vi "SMS Image Preview.vi"(7 "Calling VI Ref":refnum<vi>) -> ()   [LabVIEW 2020]
uses:
  <vilib>/Utility/miscctls.llb/LVPointTypeDef.ctl
  Hardware Configuration/Hardware Configuration Controls/Device Function.ctl
  SMS Image Preview Type Defs/SMS Image Preview Notifier Type.ctl
  SMS Image Preview Type Defs/SMS Image Preview Actions.ctl
  <vilib>/vision/Image Controls.llb/IMAQ Image.ctl
  Device Library/Cameras/Hamamatsu/Orca Flash/Orca Flash Controls/Orca Flash Actions.ctl
  Hardware Configuration/Hardware Configuration Controls/Device Type.ctl
  Device Library/Cameras/Camera Controls/Camera IMAQ Key Info.ctl
  <vilib>/vision/NI_Vision_Development_Module.lvlib
panel:
  in  "Reset Plot":bool
  out "Blink No. vs. Time":cluster{dbl[], u16[]}(graph)
  in  "Accumulate":bool
  in  "Blink Sensitivity":sgl=1.3
  in  "Image Display":bool
  in  "SMS Preview":bool
  in  "Camera ROI":bool
  in  "Camera":i32(ring) items=["Hamamatsu-Camera-Primary-0"]
  in  "Quit":bool
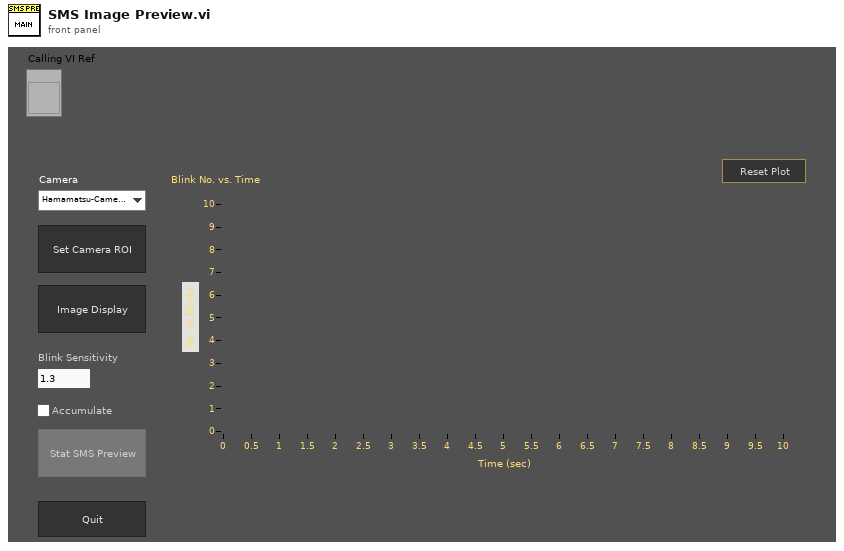
[diagram p1: front panel]
types:
  T1 = typedef "Orca Flash Actions.ctl" = enum16{"Idle", "Preview", "Record", "Record Settings", "Set Param", "Get Param", "Set ROI", "Get ROI", "Trigger Source", "Trigger Type", "Progessive Mode", "Area Mode", "Status", "Quit"}
  T2 = enum8{"Enabled", "Disabled", "Disabled and Grayed Out"}
  T3 = typedef "SMS Image Preview Actions.ctl" = enum16{"Idle", "Start SMS Preview", "Get Image", "Convolve and Threshold", "Subtract > Dilate", "And Image", "Update Plot", "Abort", "Exit Loop", "Quit"}
  T4 = typedef "SMS Image Preview Notifier Type.ctl" = cluster{"Action":T3, "Camera Notifier Name":string, "Camera Image (U16)":T5, "Camera ROI":cluster{"Global Rectangle":i32[], "Contours":cluster{"Contour Type":u32, "ROI Type":u32, "Points":i32[]}[]}, "SMS Preview (U16)":T5, "Camera ROI (U16)":T5, "Threshold (U16)":T5, "Subtracted > Dilated (U16)":T5, "And Image (U16)":T5, "Camera ROI (SGL)":T5, "Conv 5 x 5 (SGL)":T5, "Conv 11 x 11 (SGL)":T5, "Subtracted (SGL)":T5, "Dilated (SGL)":T5, "Subtracted > Dilated (SGL)":T5, "Ones 5 x 5":sgl[][], "Ones 11 x 11":sgl[][], "Ones 7 x 7":i32[][]}
  T5 = typedef "IMAQ Image.ctl" = refnum<image>
  T6 = typedef "Device Function.ctl" = enum16{"Primary", "Secondary", "Overview", "Wide Field Drift Correction", "642 nm Excitation", "560 nm Excitation", "940 nm Excitation", "546 nm Excitation", "488 nm Excitation", "405 nm Excitation", "Objective Drift Correction", "4Pi Objective Lock", "Objective XY", "Objective Z", "Sample XY", "Sample Coarse Z", "Sample Z", "4Pi Lower", "4Pi Upper", "Mojo", "Adj Cavity", "Line Scanning", "Alert"}
  T7 = enum16{"Always On", "Always Off", "Off While Running"}
  T8 = typedef "LVPointTypeDef.ctl" = cluster{"Horizontal":i16, "Vertical":i16}
  T9 = typedef "Image Type" = u32
  T10 = typedef "Device Type.ctl" = enum16{"AOTF", "Camera", "Deformable Mirror", "Laser", "Microscope Base", "Shutter", "Stage", "Waveform", "FPGA", "Email", "Filter Wheel", "Spinning Disk"}
  T11 = typedef "Camera IMAQ Key Info.ctl" = cluster{"Frame":u32, "Sensor Height":i32, "Sensor Width":i32, "ROI Height":i32, "ROI Width":i32, "ROI Enable?":bool, "Bit per Pixel":u8}
  T12 = enum32{"Average", "Min", "Max", "Clear  if < ", "Clear  if < or =", "Clear  if =", "Clear  if > or =", "Clear  if >"}
  T13 = enum32{"AutoM", "Close", "Dilate", "Erode", "Gradient", "Gradient in", "Gradient out", "HitMiss", "Open", "PClose", "POpen", "Thick", "Thin"}
  T14 = enum32{"Invalid", "Standard", "Closed", "Hidden", "Minimized", "Maximized"}
  T15 = cluster{"Global Rectangle":i32[], "Contours":cluster{"Contour Type":u32, "ROI Type":u32, "Points":i32[]}[]}
  T16 = cluster{"histogram":u32[], "Minimal Value":sgl, "Maximal Value":sgl, "Starting Value":sgl, "Interval Width":sgl, "Mean Value":sgl, "Standard  Variation":sgl, "Area (pixels)":i32}
  T17 = typedef "LVRectTypeDef.ctl" = cluster{"Left":i16, "Top":i16, "Right":i16, "Bottom":i16}
  T18 = typedef "LVBoundsTypeDef.ctl" = cluster{"Width":u32, "Height":u32}
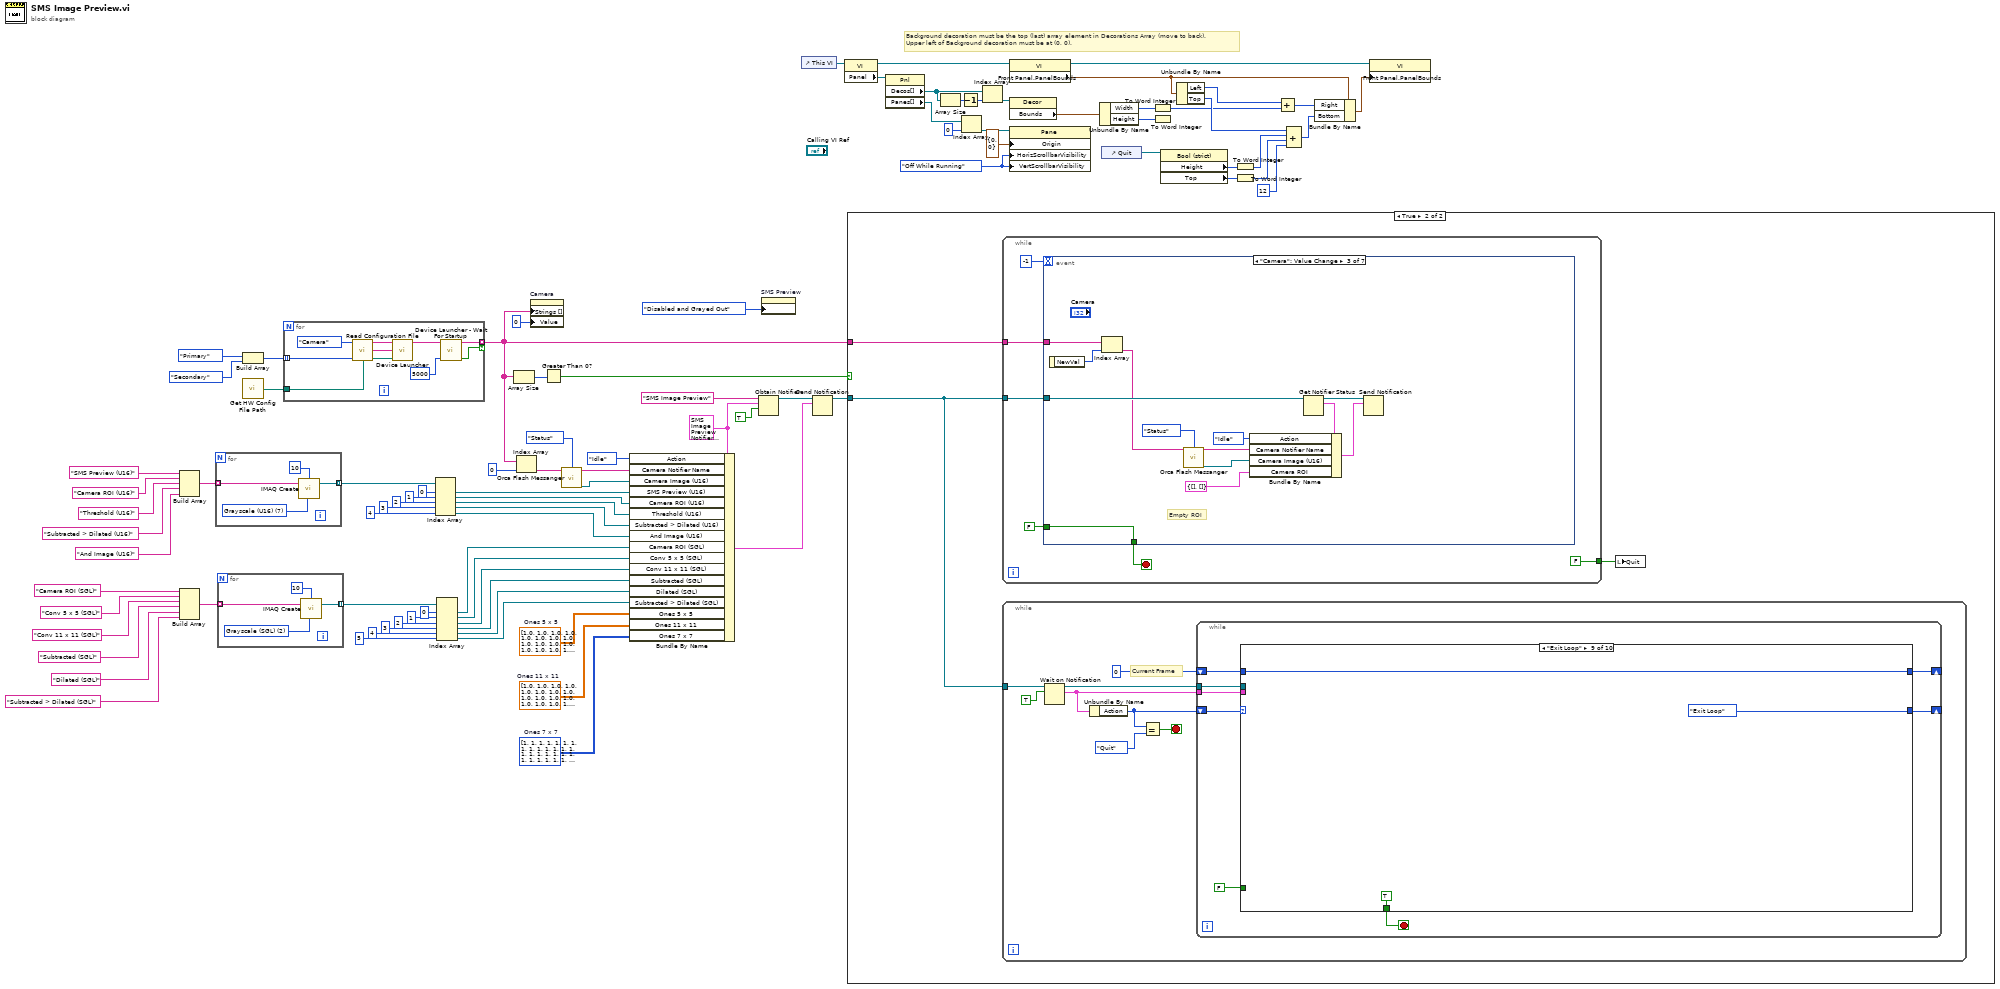
[diagram p0: block diagram]
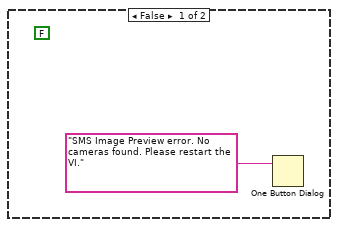
[diagram p2: hidden frame]
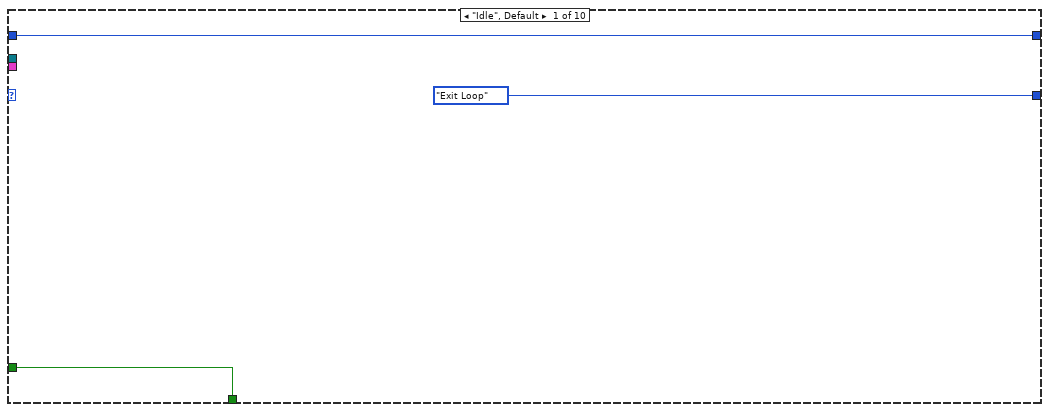
[diagram p3: hidden frame]
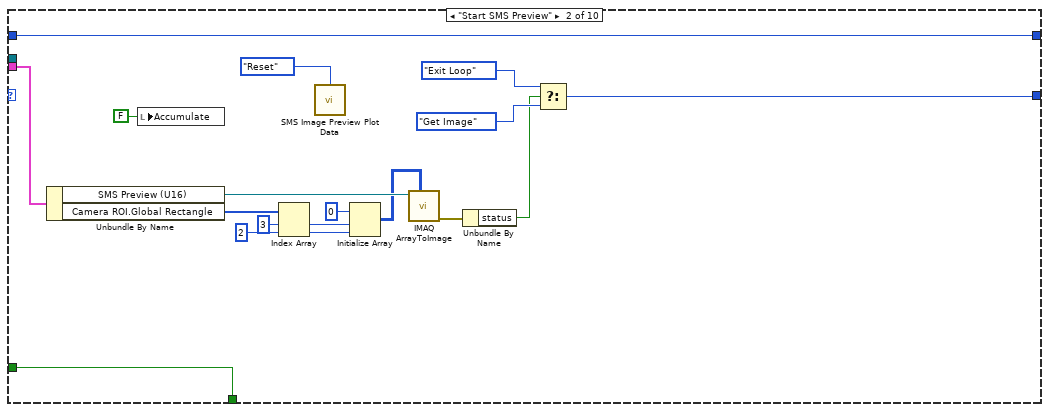
[diagram p4: hidden frame]
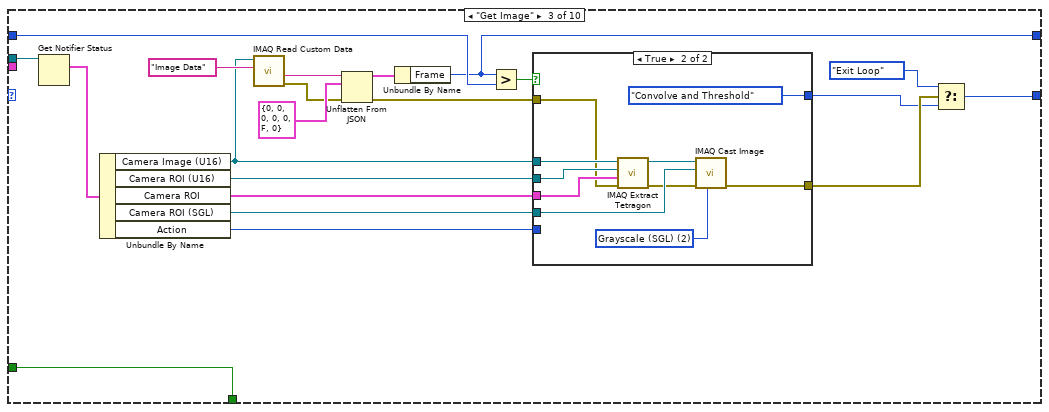
[diagram p5: hidden frame]
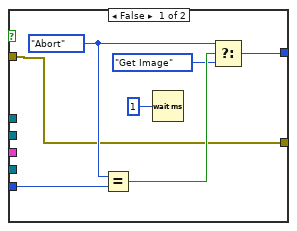
[diagram p6: hidden frame]
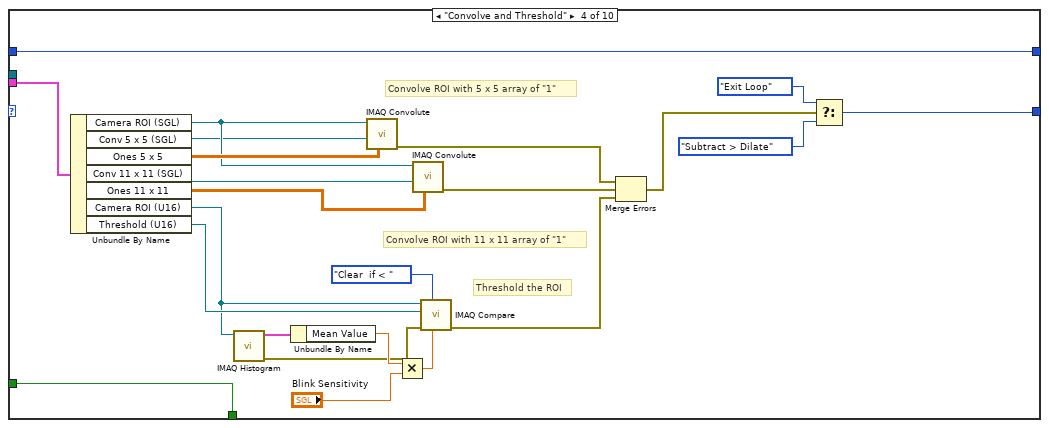
[diagram p7: hidden frame]
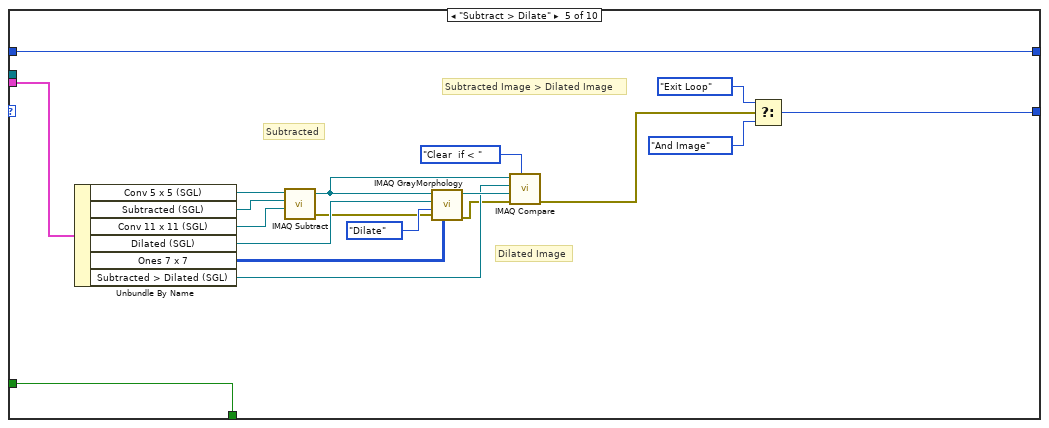
[diagram p8: hidden frame]
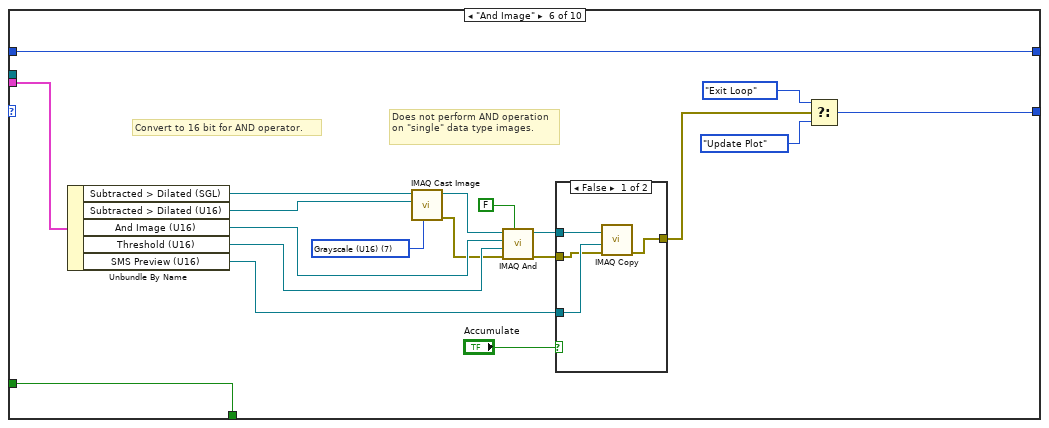
[diagram p9: hidden frame]
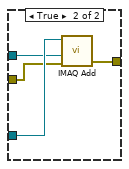
[diagram p10: hidden frame]
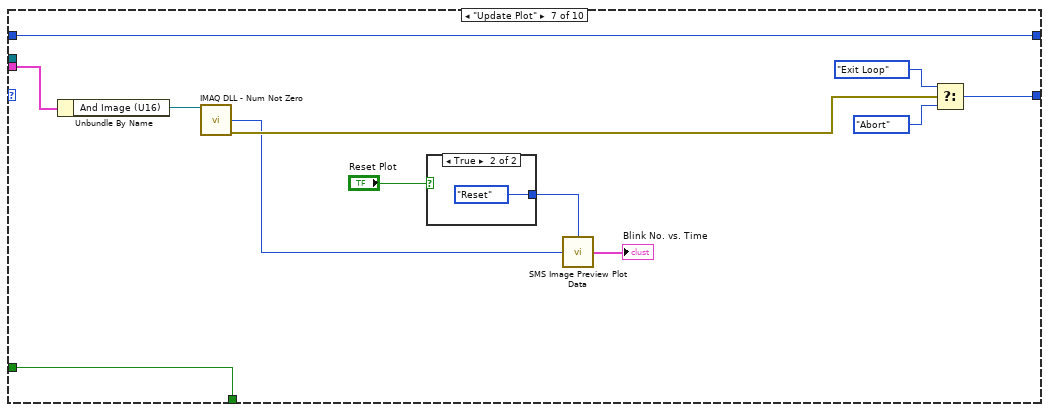
[diagram p11: hidden frame]
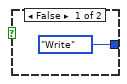
[diagram p12: hidden frame]
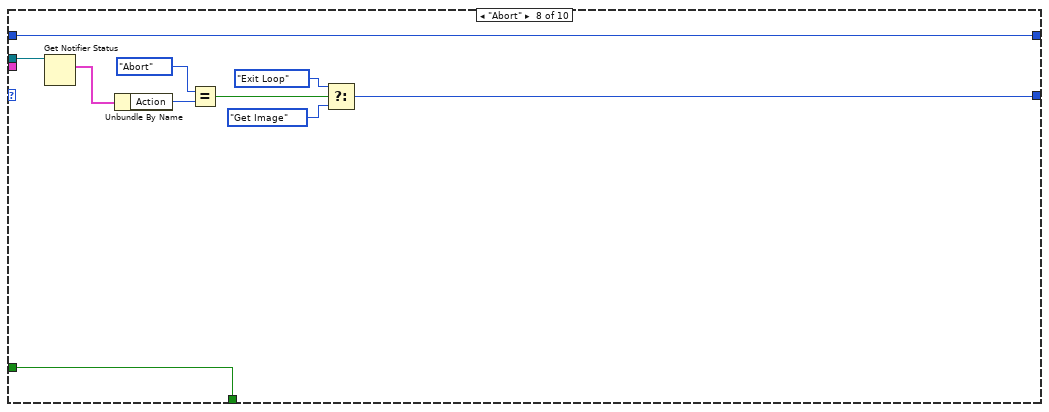
[diagram p13: hidden frame]
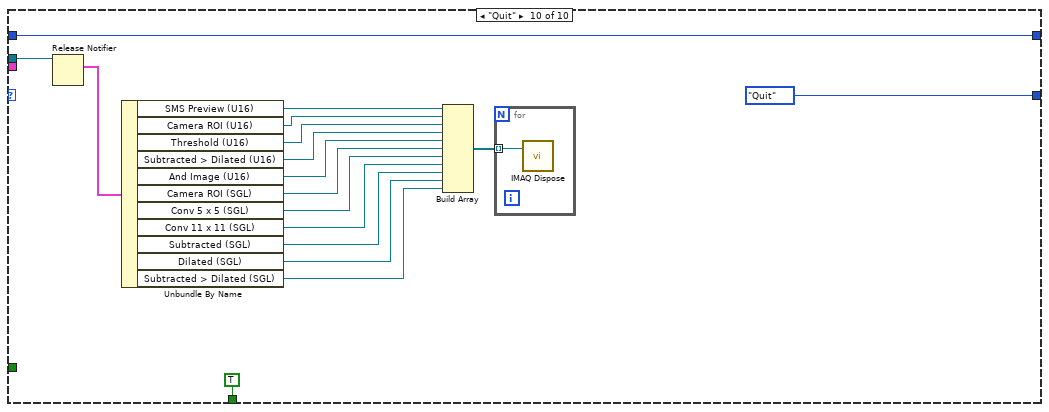
[diagram p14: hidden frame]
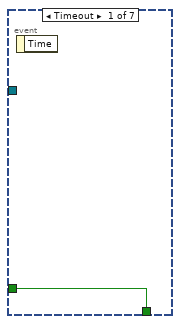
[diagram p15: hidden frame]
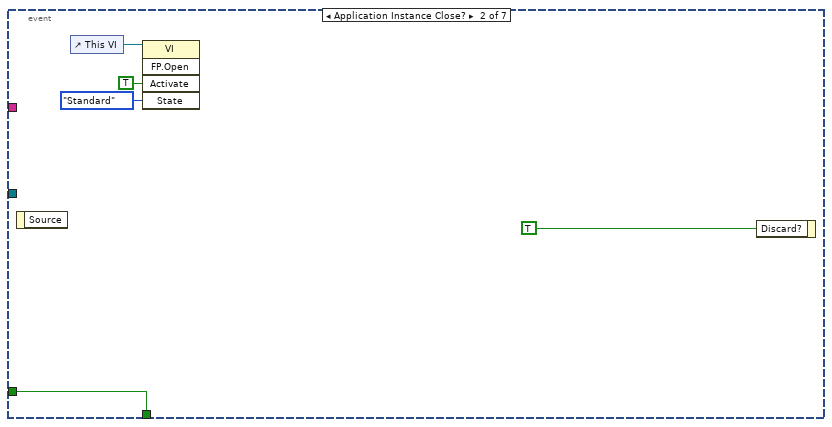
[diagram p16: hidden frame]
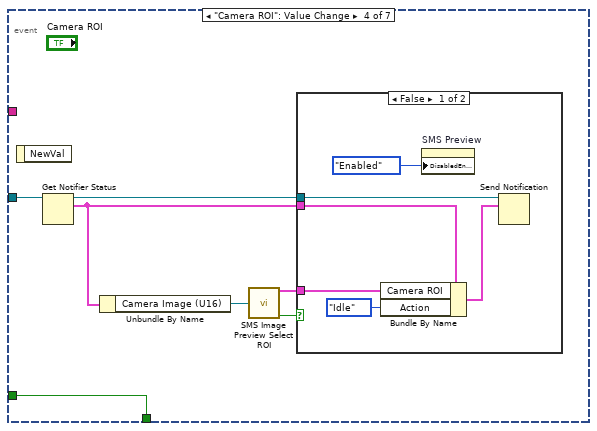
[diagram p17: hidden frame]
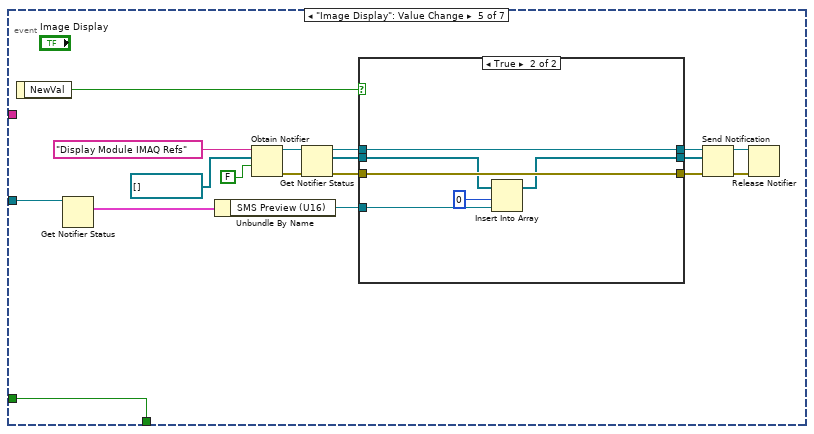
[diagram p19: hidden frame]
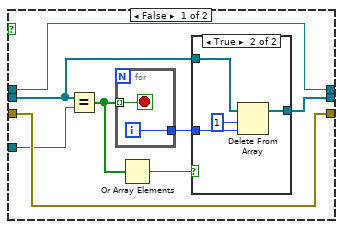
[diagram p20: hidden frame]
diagram:
  w3 = i32[][] [[1, 1, 1, 1, 1, 1, 1], [1, 1, 1, 1, 1, 1, 1], [1, 1, 1, 1, 1, 1, 1], [1, 1, 1, 1, 1, 1, 1], [1, 1, 1, 1, 1, 1, 1], [1, 1, 1, 1, 1, 1, 1], [1, 1, 1, 1, 1, 1, 1]]  # Ones 7 x 7
  w4 = sgl[][] [[1.0, 1.0, 1.0, 1.0, 1.0, 1.0, 1.0, 1.0, 1.0, 1.0, 1.0], [1.0, 1.0, 1.0, 1.0, 1.0, 1.0, 1.0, 1.0, 1.0, 1.0, 1.0], [1.0, 1.0, 1.0, 1.0, 1.0, 1.0, 1.0, 1.0, 1.0, 1.0, 1.0], [1.0, 1.0, 1.0, 1.0, 1.0, 1.0, 1.0, 1.0, 1.0, 1.0, 1.0], [1.0, 1.0, 1.0, 1.0, 1.0, 1.0, 1.0, 1.0, 1.0, 1.0, 1.0], [1.0, 1.0, 1.0, 1.0, 1.0, 1.0, 1.0, 1.0, 1.0, 1.0, 1.0], [1.0, 1.0, 1.0, 1.0, 1.0, 1.0, 1.0, 1.0, 1.0, 1.0, 1.0], [1.0, 1.0, 1.0, 1.0, 1.0, 1.0, 1.0, 1.0, 1.0, 1.0, 1.0], [1.0, 1.0, 1.0, 1.0, 1.0, 1.0, 1.0, 1.0, 1.0, 1.0, 1.0], [1.0, 1.0, 1.0, 1.0, 1.0, 1.0, 1.0, 1.0, 1.0, 1.0, 1.0], [1.0, 1.0, 1.0, 1.0, 1.0, 1.0, 1.0, 1.0, 1.0, 1.0, 1.0]]  # Ones 11 x 11
  w5 = sgl[][] [[1.0, 1.0, 1.0, 1.0, 1.0], [1.0, 1.0, 1.0, 1.0, 1.0], [1.0, 1.0, 1.0, 1.0, 1.0], [1.0, 1.0, 1.0, 1.0, 1.0], [1.0, 1.0, 1.0, 1.0, 1.0]]  # Ones 5 x 5
  w51 = T4 {"Action"=enum."Idle", "Camera Notifier Name"="", "Camera Image (U16)"=refnum, "Camera ROI"={"Global Rectangle"=[], "Contours"=[]}, "SMS Preview (U16)"=refnum, "Camera ROI (U16)"=refnum, "Threshold (U16)"=refnum, "Subtracted > Dilated (U16)"=refnum, "And Image (U16)"=refnum, "Camera ROI (SGL)"=refnum, "Conv 5 x 5 (SGL)"=refnum, "Conv 11 x 11 (SGL)"=refnum, "Subtracted (SGL)"=refnum, "Dilated (SGL)"=refnum, "Subtracted > Dilated (SGL)"=refnum, "Ones 5 x 5"=[], "Ones 11 x 11"=[], "Ones 7 x 7"=[]} ("SMS Image Preview Notifier Type")
  w73 = T7."Off While Running" ("Vertical Scrollbar Visibility")
  # "Background decoration must be the top (last) array element in Decorations Array (move to back).\nUpper left of Background decoration must be at (0, 0)."
  n1 = Build Array("Camera ROI (SGL)" ("Image Name"), "Conv 5 x 5 (SGL)" ("Image Name"), "Conv 11 x 11 (SGL)" ("Image Name"), "Subtracted (SGL)" ("Image Name"), "Dilated (SGL)" ("Image Name"), "Subtracted > Dilated (SGL)" ("Image Name")) -> (w37:string[])
  n2 = Build Array("SMS Preview (U16)" ("Image Name"), "Camera ROI (U16)" ("Image Name"), "Threshold (U16)" ("Image Name"), "Subtracted > Dilated (U16)" ("Image Name"), "And Image (U16)" ("Image Name")) -> (w17:string[])
  n3 = for {
    tunnel: w17 -> [w92] mode=indexing
    tunnel: [w91] -> w18 mode=indexing
    w93 = T9 7 items=["Grayscale (U8)", "Grayscale (I16)", "Grayscale (SGL)", "Complex (CSG)", "RGB (U32)", "HSL (U32)", "RGB (U64)", "Grayscale (U16)"] ("Image Type")
    n4 = call "IMAQ Create"("Border Size"=10, "Image Name"=w92, "Image Type"=w93) -> ("New Image"=w91:T5)  [unwired: 2 in, 1 out]
  }
  n5 = for {
    tunnel: w37 -> [w96] mode=indexing
    tunnel: [w95] -> w36 mode=indexing
    w97 = T9 2 items=["Grayscale (U8)", "Grayscale (I16)", "Grayscale (SGL)", "Complex (CSG)", "RGB (U32)", "HSL (U32)", "RGB (U64)", "Grayscale (U16)"] ("Image Type")
    n6 = call "IMAQ Create"("Border Size"=10, "Image Name"=w96, "Image Type"=w97) -> ("New Image"=w95:T5)  [unwired: 2 in, 1 out]
  }
  n7 = Build Array(Device_Function."Primary" ("Device Function"), Device_Function."Secondary" ("Device Function")) -> (w59:T6[])
  n8 = call "Get HW Config File Path.vi"() -> ("File Path"=w58:path)  [unwired: 14 in, 1 out]
  n9 = for {
    tunnel: w59 -> [w104] mode=indexing
    tunnel: w58 -> [w103]
    tunnel: [w101] -> w47 mode=indexing if=w100
    n10 = call "Read Configuration File.vi"("Device Type"=Device_Type."Camera", "Device Function"=w104, "Config File Path"=w103) -> ("Unique Notifier Name"=w106:string, "Device Ports/IDs/Channels"=w108:string[], "Device Engine Path"=w107:path)  [unwired: 9 in, 1 out]
    n11 = call "Device Launcher.vi"("Notifier Name"=w106, "Device Ports/IDs/Channels"=w108, "Device Engine Path"=w107) -> ("Notifier Name"=w102:string)  [unwired: 11 in, 1 out]
    n12 = call "Device Launcher - Wait For Startup.vi"("Notifier Name"=w102, "Wait Time (ms)"=5000) -> ("Notifier Name (Dup)"=w101:string, "Running?"=w100:bool)  [unwired: 12 in]
  }
  n13 = Index Array(array=w18, index #1=0 ("index"), index #2=1 ("index"), index #3=2 ("index"), index #4=3 ("index"), index #5=4 ("index")) -> (element #1=w16:T5, element #2=w15:T5, element #3=w14:T5, element #4=w13:T5, element #5=w12:T5)
  n14 = Index Array(array=w36, index #1=0 ("index"), index #2=1 ("index"), index #3=2 ("index"), index #4=3 ("index"), index #5=4 ("index"), index #6=5 ("index")) -> (element #1=w11:T5, element #2=w10:T5, element #3=w9:T5, element #4=w8:T5, element #5=w7:T5, element #6=w6:T5)
  n15 = Array Size(array=w47) -> (size(s)=w57:i32)
  n16 = Index Array(array=w47, index=0) -> (element=w45:string)
  n17 = property on="Camera" class="Ring (strict)"("Strings []"=w47, "Value"=0) -> ()  [unwired: 2 in, 2 out]
  n18 = Greater Than 0?(x=w57) -> (x > 0?=w56:bool)
  n19 = call "Orca Flash Messanger.vi"("Notifier Name"=w45, "Camera Actions"=Orca_Flash_Actions."Status") -> ("Notifier Name Dup"=w44:string, "Image Ref"=w43:T5)  [unwired: 9 in, 3 out]
  n20 = Bundle By Name(cluster=w51, "Action"=SMS_Image_Preview_Actions."Idle", "Camera Notifier Name"=w44, "Camera Image (U16)"=w43, "SMS Preview (U16)"=w16, "Camera ROI (U16)"=w15, "Threshold (U16)"=w14, "Subtracted > Dilated (U16)"=w13, "And Image (U16)"=w12, "Camera ROI (SGL)"=w11, "Conv 5 x 5 (SGL)"=w10, "Conv 11 x 11 (SGL)"=w9, "Subtracted (SGL)"=w8, "Dilated (SGL)"=w7, "Subtracted > Dilated (SGL)"=w6, "Ones 5 x 5"=w5, "Ones 11 x 11"=w4, "Ones 7 x 7"=w3) -> (w48:T4)
  n21 = Obtain Notifier(name (unnamed)="SMS Image Preview", notification data type=w51, create if not found? (T)=TRUE) -> (notifier out=w52:refnum<notifier>)  [unwired: 1 in, 2 out]
  n22 = property on="SMS Preview" class="Bool (strict)"("DisabledEnum"=T2."Disabled and Grayed Out" ("Disabled")) -> ()  [unwired: 2 in, 2 out]
  n23 = control-ref of="This VI"() -> (w65:refnum<vi>)
  n24 = Send Notification(notification=w48, notifier=w52) -> (notifier out=w49:refnum<notifier>)  [unwired: 1 in, 1 out]
  n25 = property class="VI"(reference=w65) -> (reference out=w74:refnum<vi>, "Panel"=w66:refnum<vi>)  [unwired: 1 in, 1 out]
  n26 = case shown="True" w56 {
    tunnel: w47 -> [_ w112]
    tunnel: w49 -> [_ w110]
    frame False {
      (unwired) FALSE
      n27 = One Button Dialog(message="SMS Image Preview error. No cameras found. Please restart the VI.") -> ()  [unwired: 1 in, 1 out]
    }
    frame True {
      n28 = while {
        tunnel: w112 -> [w304]
        tunnel: w110 -> [w303]
        tunnel: [FALSE] -> w111
        stop <- w305 stop-if-true
        n29 = event shown="[2] \"Camera\": Value Change" {
          selector: _ -> [_ _ _ _ _ _ _]
          dyn-events: _ -> [_ _ _ _ _ _ _]
          timeout: -1 -> [_ _ _ _ _ _ _]
          tunnel: FALSE -> [w308 w312 w326 w333 w357 w387 _]
          tunnel: [w308 w312 w326 w333 w357 w387 w393] -> w305
          tunnel: w304 -> [_ _ w325 _ _ _ _]
          tunnel: w303 -> [_ _ w323 w332 w341 w386 w392]
          event Timeout {
            n30 = event-data() -> ()  [unwired: 1 in, 1 out]
          }
          event Application Instance Close? {
            n31 = event-data() -> ()  [unwired: 1 in, 1 out]
            n32 = control-ref of="This VI"() -> (w309:refnum<vi>)
            n33 = invoke class="VI" method="FP.Open"(reference=w309, "Activate"=TRUE ("Activate?"), "State"=T14."Standard") -> ()  [unwired: 2 in, 5 out]
            n34 = event-data("Discard?"=TRUE) -> ()  [unwired: 1 in, 1 out]
          }
          event "Camera": Value Change {
            # "Empty ROI"
            n35 = event-data() -> ("NewVal"=w324:i32)  [unwired: 1 in]
            n36 = Index Array(array=w325, index=w324) -> (element=w317:string)
            n37 = call "Orca Flash Messanger.vi"("Notifier Name"=w317, "Camera Actions"=Orca_Flash_Actions."Status") -> ("Notifier Name Dup"=w319:string, "Image Ref"=w318:T5)  [unwired: 9 in, 3 out]
            n38 = Get Notifier Status(notifier=w323) -> (notifier out=w322:refnum<notifier>, current notification=w321:T4)  [unwired: 1 in, 3 out]
            n39 = Bundle By Name(cluster=w321, "Action"=SMS_Image_Preview_Actions."Idle", "Camera Notifier Name"=w319, "Camera Image (U16)"=w318, "Camera ROI"=T15 {"Global Rectangle"=[], "Contours"=[]}) -> (w320:T4)
            n40 = Send Notification(notification=w320, notifier=w322) -> ()  [unwired: 1 in, 2 out]
          }
          event "Camera ROI": Value Change {
            n41 = event-data() -> ()  [unwired: 1 in, 1 out]
            n42 = Get Notifier Status(notifier=w332) -> (notifier out=w331:refnum<notifier>, current notification=w327:T4)  [unwired: 1 in, 3 out]
            n43 = Unbundle By Name(w327) -> ("Camera Image (U16)"=w330:T5)
            n44 = call "SMS Image Preview Select ROI.vi"("Camera Image Ref"=w330) -> ("Camera ROI"=w328:T15, "Canceled?"=w329:bool)  [unwired: 13 in]
            n45 = case shown="False" w329 {
              tunnel: w331 -> [w339 _]
              tunnel: w328 -> [w337 _]
              tunnel: w327 -> [w338 _]
              frame False {
                n46 = Bundle By Name(cluster=w338, "Camera ROI"=w337, "Action"=SMS_Image_Preview_Actions."Idle") -> (w336:T4)
                n47 = property on="SMS Preview" class="Bool (strict)"("DisabledEnum"=T2."Enabled" ("Disabled")) -> ()  [unwired: 2 in, 2 out]
                n48 = Send Notification(notification=w336, notifier=w339) -> ()  [unwired: 1 in, 2 out]
              }
              frame True {
              }
            }
          }
          event "Image Display": Value Change {
            n49 = event-data() -> ("NewVal"=w340:bool)  [unwired: 1 in]
            n50 = Get Notifier Status(notifier=w341) -> (current notification=w342:T4)  [unwired: 1 in, 4 out]
            n51 = Unbundle By Name(w342) -> ("SMS Preview (U16)"=w356:T5)
            n52 = Obtain Notifier(name (unnamed)="Display Module IMAQ Refs", notification data type=T5[] [], create if not found? (T)=FALSE) -> (notifier out=w349:refnum<notifier>, error out=w350:errorcluster)  [unwired: 1 in, 1 out]
            n53 = Get Notifier Status(notifier=w349, error in (no error)=w350) -> (notifier out=w348:refnum<notifier>, current notification=w346:T5[], error out=w347:errorcluster)  [unwired: 2 out]
            n54 = case shown="True" w340 {
              tunnel: w348 -> [w365 w378]
              tunnel: w347 -> [w359 w377]
              tunnel: w346 -> [w361 w376]
              tunnel: [w360 w373] -> w343
              tunnel: [w365 w378] -> w345
              tunnel: [w359 w377] -> w344
              tunnel: w356 -> [w358 w375]
              frame False {
                n55 = Equal?(x=w361, y=w358) -> (x = y?=w364:bool[])
                n56 = for {
                  tunnel: w364 -> [w372] mode=indexing
                  tunnel: [w371] -> w362
                  i -> [w371]
                  stop <- w372 stop-if-true
                }
                n57 = Or Array Elements(Boolean array=w364) -> (logical OR=w363:bool)
                n58 = case shown="True" w363 {
                  tunnel: w362 -> [_ w369]
                  tunnel: w361 -> [w366 w368]
                  tunnel: [w366 w367] -> w360
                  frame False {
                  }
                  frame True {
                    n59 = Delete From Array(array=w368, length=1, index=w369) -> (array with subset deleted=w367:T5[])  [unwired: 1 out]
                  }
                }
              }
              frame True {
                n60 = Insert Into Array(array=w376, index=0, new element=w375) -> (w373:T5[])
              }
            }
            n61 = Send Notification(notification=w343, notifier=w345, error in (no error)=w344) -> (notifier out=w351:refnum<notifier>, error out=w352:errorcluster)
            n62 = Release Notifier(notifier=w351, error in (no error)=w352) -> ()  [unwired: 1 in, 3 out]
          }
          event "SMS Preview": Value Change {
            n63 = event-data() -> ("NewVal"=w382:bool)  [unwired: 1 in]
            n64 = Get Notifier Status(notifier=w386) -> (notifier out=w385:refnum<notifier>, current notification=w384:T4)  [unwired: 1 in, 3 out]
            n65 = Select(t=SMS_Image_Preview_Actions."Start SMS Preview" ("Action"), s=w382, f=SMS_Image_Preview_Actions."Abort") -> (s? t:f=w379:T3)
            n66 = Bundle By Name(cluster=w384, "Action"=w379) -> (w383:T4)
            n67 = Send Notification(notification=w383, notifier=w385) -> ()  [unwired: 1 in, 2 out]
          }
          event "Quit": Value Change {
            n68 = event-data() -> ("NewVal"=w393:bool)  [unwired: 1 in]
            n69 = Get Notifier Status(notifier=w392) -> (notifier out=w390:refnum<notifier>, current notification=w389:T4)  [unwired: 1 in, 3 out]
            n70 = Bundle By Name(cluster=w389, "Action"=SMS_Image_Preview_Actions."Quit") -> (w391:T4)
            n71 = Send Notification(notification=w391, notifier=w390) -> ()  [unwired: 1 in, 2 out]
          }
        }
      }
      n72 = while {
        tunnel: w110 -> [w120]
        stop <- w117 stop-if-true
        # "Current Frame"
        n73 = Wait on Notification(notifier=w120, ignore previous (F)=TRUE) -> (notifier out=w113:refnum<notifier>, notification=w115:T4)  [unwired: 2 in, 2 out]
        n74 = Unbundle By Name(w115) -> ("Action"=w116:T3)
        n75 = Equal?(x=w116, y=SMS_Image_Preview_Actions."Quit") -> (x = y?=w117:bool)
        n76 = while {
          shift-right: [w126] -> _
          shift-left: w116 -> [w128]
          tunnel: w115 -> [w127]
          shift-right: [w124] -> _
          shift-left: u32 0 -> [w125]
          tunnel: w113 -> [w123]
          stop <- w121 stop-if-true
          n77 = case shown="\"Exit Loop\"" w128 {
            tunnel: w127 -> [_ w147 _ w209 w228 w247 w263 _ _ _]
            tunnel: [SMS_Image_Preview_Actions."Exit Loop" ("y") w136 w151 w190 w211 w230 w266 w274 SMS_Image_Preview_Actions."Exit Loop" ("f") SMS_Image_Preview_Actions."Quit" ("f")] -> w126
            tunnel: w125 -> [w130 w149 w166 w210 w229 w248 w267 w280 w283 w300]
            tunnel: [w130 w149 w165 w210 w229 w248 w267 w280 w283 w300] -> w124
            tunnel: w123 -> [_ _ w159 _ _ _ _ w279 _ w297]
            tunnel: FALSE -> [w129 w148 w160 w200 w217 w237 w268 w272 _ _]
            tunnel: [w129 w148 w160 w200 w217 w237 w268 w272 TRUE TRUE] -> w121
            frame "Idle", Default {
            }
            frame "Start SMS Preview" {
              n78 = Unbundle By Name(w147) -> ("SMS Preview (U16)"=w140:T5, "Camera ROI.Global Rectangle"=w146:i32[])
              n79 = local write "Accumulate"(FALSE ("Accumulate")) -> ()
              n80 = Index Array(array=w146, index #1=3 ("index"), index #2=2 ("index")) -> (element #1=w142:i32, element #2=w141:i32)
              n81 = call "SMS Image Preview Plot Data.vi"("Plot Data Actions"=enum16{"Read", "Write", "Reset"}."Reset") -> ()  [unwired: 14 in, 1 out]
              n82 = Initialize Array(u16 0 ("index"), w142, w141) -> (w139:u16[][])
              n83 = call "IMAQ ArrayToImage"("Image Pixels (U16)"=w139, "Image"=w140) -> ("error out"=w138:errorcluster)  [unwired: 8 in, 1 out]
              n84 = Unbundle By Name(w138) -> ("status"=w135:bool)
              n85 = Select(t=SMS_Image_Preview_Actions."Exit Loop", s=w135, f=SMS_Image_Preview_Actions."Get Image" ("y")) -> (s? t:f=w136:T3)
            }
            frame "Get Image" {
              n86 = Get Notifier Status(notifier=w159) -> (current notification=w158:T4)  [unwired: 1 in, 4 out]
              n87 = Unbundle By Name(w158) -> ("Camera Image (U16)"=w163:T5, "Camera ROI (U16)"=w162:T5, "Camera ROI"=w161:T15, "Camera ROI (SGL)"=w156:T5, "Action"=w157:T3)
              n88 = call "IMAQ Read Custom Data"("Key"="Image Data", "Image"=w163) -> ("error out"=w155:errorcluster, "Custom Data Out"=w168:string)  [unwired: 7 in, 1 out]
              n89 = Unflatten From JSON(JSON string=w168, type and defaults=T11 {"Frame"=0, "Sensor Height"=0, "Sensor Width"=0, "ROI Height"=0, "ROI Width"=0, "ROI Enable?"=FALSE, "Bit per Pixel"=0} ("Camera IMAQ Key Info"), error in (no error)=w155) -> (value=w170:T11, error out=w154:errorcluster)  [unwired: 4 in]
              n90 = Unbundle By Name(w170) -> ("Frame"=w165:u32)
              n91 = Greater?(x=w165, y=w166) -> (0:w164:bool)
              n92 = case shown="True" w164 {
                tunnel: w163 -> [_ w187]
                tunnel: w162 -> [_ w186]
                tunnel: w161 -> [_ w185]
                tunnel: [w175 SMS_Image_Preview_Actions."Convolve and Threshold" ("y")] -> w152
                tunnel: w157 -> [w177 _]
                tunnel: w156 -> [_ w181]
                tunnel: w154 -> [w171 w180]
                tunnel: [w171 w178] -> w153
                frame False {
                  w176 = SMS_Image_Preview_Actions."Abort" ("x")
                  n93 = Equal?(x=w176, y=w177) -> (x = y?=w174:bool)
                  n94 = Wait (ms)(milliseconds to wait=u32 1) -> ()  [unwired: 1 out]
                  n95 = Select(t=w176, s=w174, f=SMS_Image_Preview_Actions."Get Image" ("y")) -> (s? t:f=w175:T3)
                }
                frame True {
                  w183 = T9 2 items=["Grayscale (U8)", "Grayscale (I16)", "Grayscale (SGL)", "Complex (CSG)", "RGB (U32)", "HSL (U32)", "RGB (U64)", "Grayscale (U16)"] ("Image Type")
                  n96 = call-poly "IMAQ Extract Tetragon"("error in (no error)"=w180, "ROI Descriptor"=w185, "Image Dst"=w186, "Image Src"=w187) -> ("error out"=w179:errorcluster, "Image Dst Out"=w182:T5)  [unwired: 6 in]
                  n97 = call "IMAQ Cast Image"("Image Type"=w183, "error in (no error)"=w179, "Image Dst"=w181, "Image Src"=w182) -> ("error out"=w178:errorcluster)  [unwired: 6 in, 1 out]
                }
              }
              n98 = Select(t=SMS_Image_Preview_Actions."Exit Loop", s=w153, f=w152) -> (s? t:f=w151:T3)
            }
            frame "Convolve and Threshold" {
              # "Threshold the ROI"
              # "Convolve ROI with 11 x 11 array of \"1\""
              # "Convolve ROI with 5 x 5 array of \"1\""
              n99 = Unbundle By Name(w209) -> ("Camera ROI (SGL)"=w202:T5, "Conv 5 x 5 (SGL)"=w199:T5, "Ones 5 x 5"=w208:sgl[][], "Conv 11 x 11 (SGL)"=w198:T5, "Ones 11 x 11"=w207:sgl[][], "Camera ROI (U16)"=w197:T5, "Threshold (U16)"=w201:T5)
              n100 = call "IMAQ Histogram"("Image"=w197) -> ("error out"=w188:errorcluster, "Histogram Report"=w204:T16)  [unwired: 9 in]
              n101 = Unbundle By Name(w204) -> ("Mean Value"=w205:sgl)
              n102 = call "IMAQ Convolute"("Kernel"=w208, "Image Dst"=w199, "Image Src"=w202) -> ("error out"=w195:errorcluster)  [unwired: 7 in, 1 out]
              n103 = Multiply(x=w205, y="Blink Sensitivity") -> (x*y=w206:sgl)
              n104 = call "IMAQ Convolute"("Kernel"=w207, "Image Dst"=w198, "Image Src"=w202) -> ("error out"=w194:errorcluster)  [unwired: 7 in, 1 out]
              n105 = call "IMAQ Compare"("Constant"=w206, "Operator"=T12."Clear  if < ", "error in (no error)"=w188, "Image Dst"=w201, "Image Src A"=w197) -> ("error out"=w193:errorcluster)  [unwired: 5 in, 1 out]
              n106 = Merge Errors(w195, w194, w193) -> (w192:errorcluster)
              n107 = Select(t=SMS_Image_Preview_Actions."Exit Loop", s=w192, f=SMS_Image_Preview_Actions."Subtract > Dilate" ("y")) -> (s? t:f=w190:T3)
            }
            frame "Subtract > Dilate" {
              # "Subtracted Image > Dilated Image"
              # "Subtracted"
              # "Dilated Image"
              n108 = Unbundle By Name(w228) -> ("Conv 5 x 5 (SGL)"=w227:T5, "Subtracted (SGL)"=w226:T5, "Conv 11 x 11 (SGL)"=w225:T5, "Dilated (SGL)"=w222:T5, "Ones 7 x 7"=w223:i32[][], "Subtracted > Dilated (SGL)"=w218:T5)
              n109 = call "IMAQ Subtract"("Image Src A"=w227, "Image Dst"=w226, "Image Src B"=w225) -> ("Image Dst Out"=w219:T5, "error out"=w216:errorcluster)  [unwired: 4 in]
              n110 = call "IMAQ GrayMorphology"("Structuring Element"=w223, "error in (no error)"=w216, "Operation"=T13."Dilate", "Image Dst"=w222, "Image Src"=w219) -> ("error out"=w215:errorcluster, "Image Dst Out"=w220:T5)  [unwired: 5 in]
              n111 = call "IMAQ Compare"("Operator"=T12."Clear  if < ", "error in (no error)"=w215, "Image Src B"=w220, "Image Dst"=w218, "Image Src A"=w219) -> ("error out"=w214:errorcluster)  [unwired: 5 in, 1 out]
              n112 = Select(t=SMS_Image_Preview_Actions."Exit Loop", s=w214, f=SMS_Image_Preview_Actions."And Image" ("y")) -> (s? t:f=w211:T3)
            }
            frame "And Image" {
              w245 = T9 7 items=["Grayscale (U8)", "Grayscale (I16)", "Grayscale (SGL)", "Complex (CSG)", "RGB (U32)", "HSL (U32)", "RGB (U64)", "Grayscale (U16)"] ("Image Type")
              # "Convert to 16 bit for AND operator."
              # "Does not perform AND operation on \"single\" data type images."
              n113 = Unbundle By Name(w247) -> ("Subtracted > Dilated (SGL)"=w244:T5, "Subtracted > Dilated (U16)"=w243:T5, "And Image (U16)"=w241:T5, "Threshold (U16)"=w240:T5, "SMS Preview (U16)"=w238:T5)
              n114 = call "IMAQ Cast Image"("Image Type"=w245, "Image Dst"=w243, "Image Src"=w244) -> ("error out"=w235:errorcluster, "Image Dst Out"=w242:T5)  [unwired: 7 in]
              n115 = call "IMAQ And"("And/Nand (And)"=FALSE, "error in (no error)"=w235, "Image Src B"=w240, "Image Dst"=w241, "Image Src A"=w242) -> ("error out"=w234:errorcluster, "Image Dst Out"=w239:T5)  [unwired: 5 in]
              n116 = case shown="False" "Accumulate" {
                tunnel: w239 -> [w252 w255]
                tunnel: w238 -> [w251 w256]
                tunnel: w234 -> [w250 w254]
                tunnel: [w249 w253] -> w231
                frame False {
                  n117 = call "IMAQ Copy"("error in (no error)"=w250, "Image Dst"=w251, "Image Src"=w252) -> ("error out"=w249:errorcluster)  [unwired: 3 in, 1 out]
                }
                frame True {
                  n118 = call "IMAQ Add"("Image Src A"=w256, "Image Src B"=w255, "error in (no error)"=w254) -> ("error out"=w253:errorcluster)  [unwired: 4 in, 1 out]
                }
              }
              n119 = Select(t=SMS_Image_Preview_Actions."Exit Loop", s=w231, f=SMS_Image_Preview_Actions."Update Plot" ("y")) -> (s? t:f=w230:T3)
            }
            frame "Update Plot" {
              n120 = Unbundle By Name(w263) -> ("And Image (U16)"=w262:T5)
              n121 = call "IMAQ DLL - Num Not Zero.vi"("IMAQ Ref"=w262) -> ("Non Zero Px Total"=w259:u16, "Error Out"=w261:errorcluster)  [unwired: 12 in, 1 out]
              n122 = case shown="True" "Reset Plot" {
                tunnel: [enum16{"Read", "Write", "Reset"}."Write" ("Plot Data Actions") enum16{"Read", "Write", "Reset"}."Reset" ("Plot Data Actions")] -> w260
                frame False {
                }
                frame True {
                }
              }
              n123 = call "SMS Image Preview Plot Data.vi"("Plot Data Actions"=w260, "Blink Number"=w259) -> ("Plot Data"=→"Blink No. vs. Time":cluster{dbl[], u16[]})  [unwired: 13 in]
              n124 = Select(t=SMS_Image_Preview_Actions."Exit Loop" ("y"), s=w261, f=SMS_Image_Preview_Actions."Abort" ("y")) -> (s? t:f=w266:T3)
            }
            frame "Abort" {
              n125 = Get Notifier Status(notifier=w279) -> (current notification=w278:T4)  [unwired: 1 in, 4 out]
              n126 = Unbundle By Name(w278) -> ("Action"=w277:T3)
              n127 = Equal?(x=SMS_Image_Preview_Actions."Abort" ("y"), y=w277) -> (x = y?=w273:bool)
              n128 = Select(t=SMS_Image_Preview_Actions."Exit Loop", s=w273, f=SMS_Image_Preview_Actions."Get Image") -> (s? t:f=w274:T3)
            }
            frame "Exit Loop" {
            }
            frame "Quit" {
              n129 = Release Notifier(notifier=w297) -> (last notification=w296:T4)  [unwired: 2 in, 2 out]
              n130 = Unbundle By Name(w296) -> ("SMS Preview (U16)"=w295:T5, "Camera ROI (U16)"=w293:T5, "Threshold (U16)"=w292:T5, "Subtracted > Dilated (U16)"=w291:T5, "And Image (U16)"=w290:T5, "Camera ROI (SGL)"=w289:T5, "Conv 5 x 5 (SGL)"=w288:T5, "Conv 11 x 11 (SGL)"=w287:T5, "Subtracted (SGL)"=w286:T5, "Dilated (SGL)"=w285:T5, "Subtracted > Dilated (SGL)"=w284:T5)
              n131 = Build Array(w295, w293, w292, w291, w290, w289, w288, w287, w286, w285, w284) -> (w294:T5[])
              n132 = for {
                tunnel: w294 -> [w301] mode=indexing
                n133 = call "IMAQ Dispose"("Image"=w301) -> ()  [unwired: 5 in, 1 out]
              }
            }
          }
        }
      }
      n134 = local write "Quit"(w111) -> ()
    }
  }
  n135 = property class="Pnl"(reference=w66) -> ("Decos[]"=w64:refnum<vi>[], "Panes[]"=w70:refnum<vi>[])  [unwired: 1 in, 2 out]
  n136 = Array Size(array=w64) -> (size(s)=w62:i32)
  n137 = Decrement(x=w62) -> (x-1=w63:i32)
  n138 = Index Array(array=w70, index=0) -> (element=w69:refnum<vi>)
  n139 = Index Array(array=w64, index=w63) -> (element=w72:refnum<vi>)
  n140 = property class="VI"(reference=w74) -> (reference out=w76:refnum<vi>, "Front Panel.PanelBounds"=w77:T17)  [unwired: 1 in, 1 out]
  n141 = property class="Decor"(reference=w72) -> ("Bounds"=w75:T18)  [unwired: 1 in, 2 out]
  n142 = property class="Pane"(reference=w69, "Origin"=T8 {"Horizontal"=0, "Vertical"=0}, "HorizScrollbarVisibility"=w73, "VertScrollbarVisibility"=w73) -> ()  [unwired: 1 in, 2 out]
  n143 = Unbundle By Name(w75) -> ("Width"=w80:u32, "Height"=w83:u32)
  n144 = control-ref of="Quit"() -> (w67:refnum<vi>)
  n145 = To Word Integer(number=w80) -> (16bit integer=w82:i16)
  n146 = To Word Integer(number=w83) -> ()  [unwired: 1 out]
  n147 = property class="Bool (strict)"(reference=w67) -> ("Height"=w85:u32, "Top"=w86:i32)  [unwired: 1 in, 2 out]
  n148 = Unbundle By Name(w77) -> ("Left"=w79:i16, "Top"=w90:i16)
  n149 = To Word Integer(number=w85) -> (16bit integer=w88:i16)
  n150 = To Word Integer(number=w86) -> (16bit integer=w89:i16)
  n151 = Add(x=w79, y=w82) -> (x+y=w81:i16)
  n152 = Compound Arithmetic op=ADD(w90, w88, w89, i16 12 ("y")) -> (w84:i16)
  n153 = Bundle By Name(cluster=w77, "Right"=w81, "Bottom"=w84) -> (w78:T17)
  n154 = property class="VI"(reference=w76, "Front Panel.PanelBounds"=w78) -> ()  [unwired: 1 in, 2 out]
